vi "Main.vi"() -> ()   [LabVIEW 2020]
doc: "This template is for the Queued Message Handler design pattern.\n\nThe Event Handling Loop generates messages based on user interface actions.\n\nThe Message Handling Loop processes messages generated by the Event Handling Loop, or by other messages. The messages are string values, so new messages can be added easily to the Message Cases case structure in the Message Handling Loop. Each message cluster can also provide an optional value for Message Data, which is a variant that can be converted to whatever message-specific data is required."
uses:
  controls/Parametros.ctl
  controls/UI Data.ctl
  support/Message Queue/Enqueue Message (Single).vi
  <vilib>/Utility/error.llb/Error Cluster From Error Code.vi
  <vilib>/ErrorRing/Error Ring.xnode
  support/Message Queue/Message Queue.lvlib
  support/User Event - Stop/User Event - Stop.lvlib
panel:
  out "Waveform Graph - Dark":dbl[](graph)
  in  "Exit":bool
  in  "Time unit":enum16{"Hours", "Minutes", "Seconds"}(ring)
  in  "Timeout for saving":u32
  in  "Save Switch":bool
  in  "Fecha de inicio":timestamp format="%<%.0X %x>T"
  in  "Graph Button":bool
  in  "Parámetro":T1
  in  "Temperatura carcasa":dbl
  in  "Corriente":dbl
  in  "Voltaje":dbl
  in  "Velocidad del motor":dbl
  in  "Factor de potencia":dbl
  in  "Temperatura balero":dbl
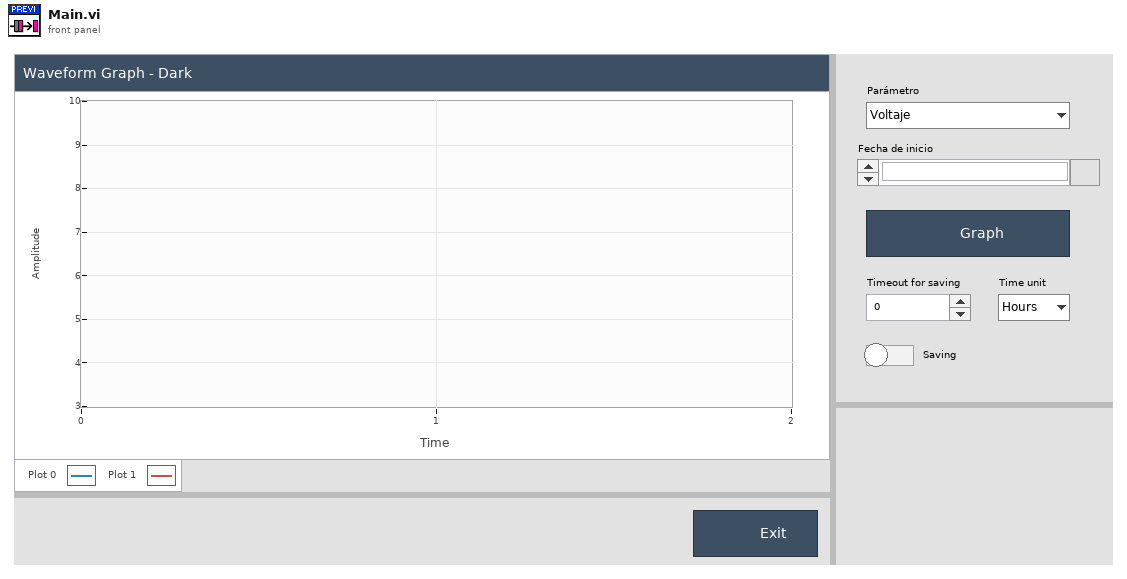
[diagram p1: front panel]
types:
  T1 = typedef "Parametros.ctl" = enum16{"Voltaje", "Corriente", "Temperatura de la carcasa", "Temperatura de balero", "Factor de potencia", "Velocidad de motor"}
  T2 = typedef "UI Data.ctl" = cluster{"Saving":bool, "Exit Button Ref":refnum<vi>, "Time":u32}
  T3 = typedef "Message Queue.lvlib/All Message Queues.ctl" = cluster{"UI":refnum<queue>}
  T4 = cluster{"Timeout for saving":u32, "Time unit":enum16{"Hours", "Minutes", "Seconds"}, "Save Switch":bool}
  T5 = cluster{"Fecha de inicio":timestamp, "Parámetro":T1}
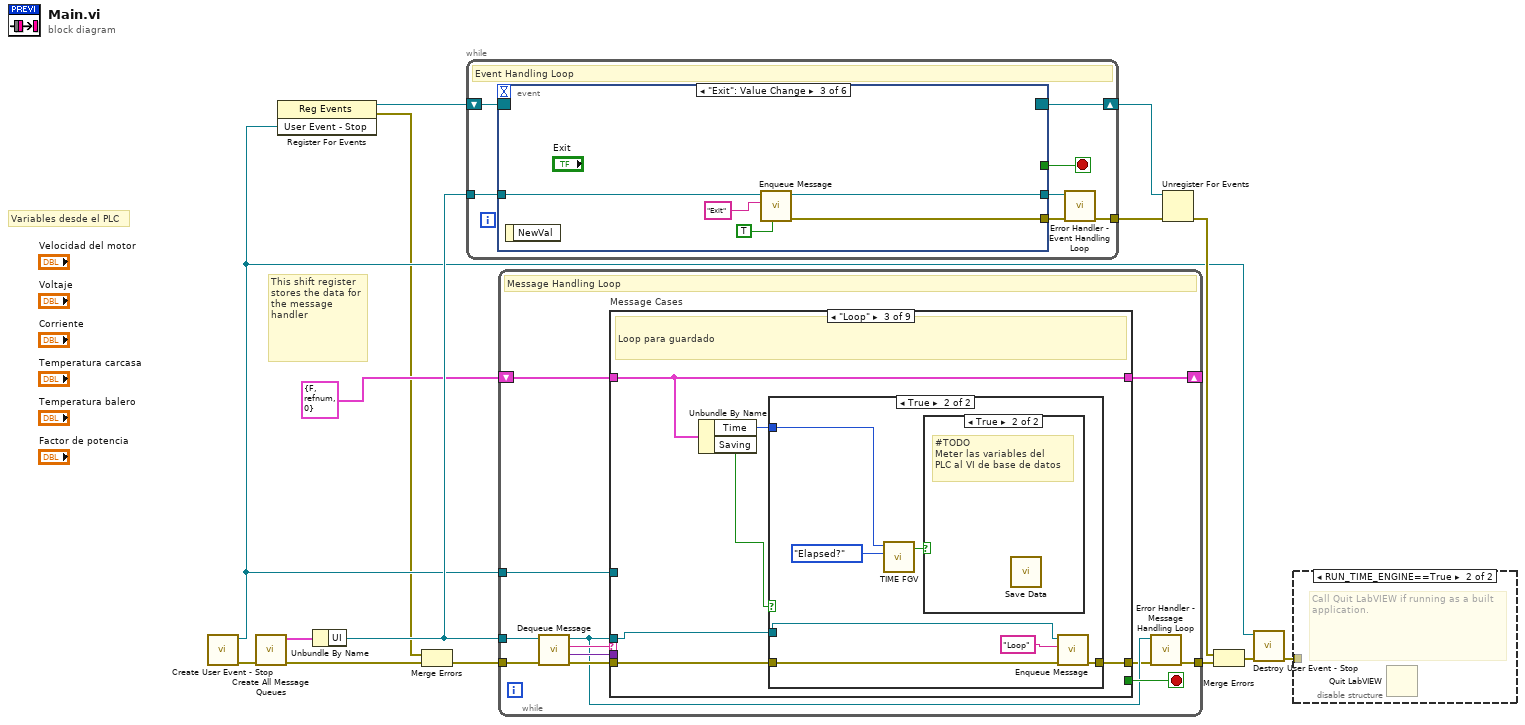
[diagram p0: block diagram]
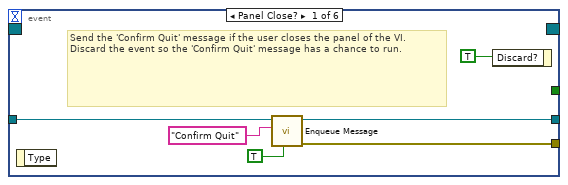
[diagram p3: hidden frame]
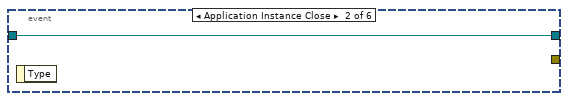
[diagram p4: hidden frame]
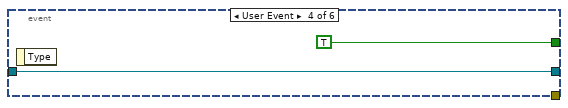
[diagram p5: hidden frame]
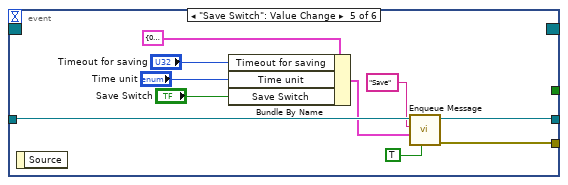
[diagram p6: hidden frame]
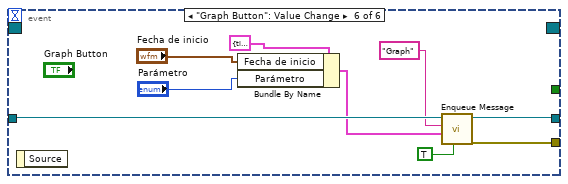
[diagram p7: hidden frame]
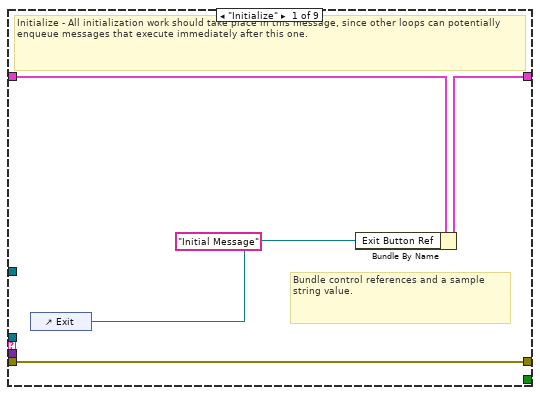
[diagram p8: hidden frame]
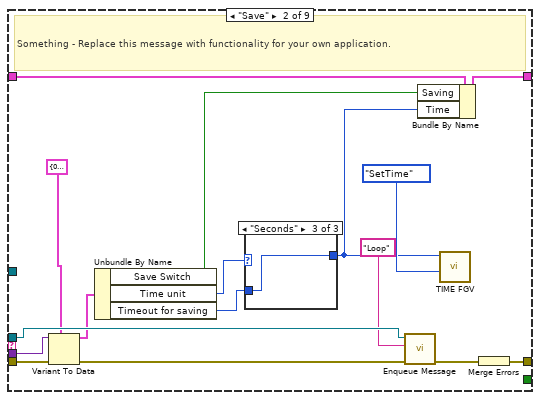
[diagram p9: hidden frame]
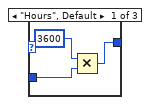
[diagram p10: hidden frame]
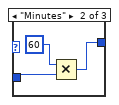
[diagram p11: hidden frame]
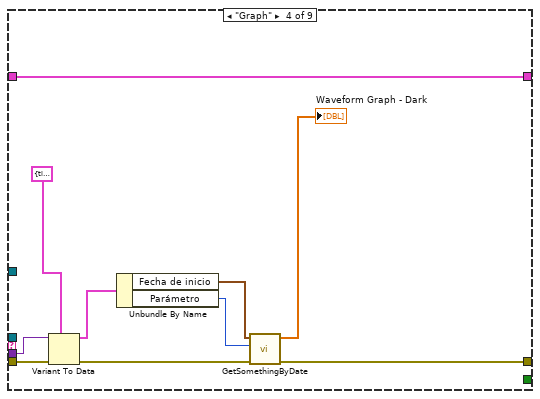
[diagram p14: hidden frame]
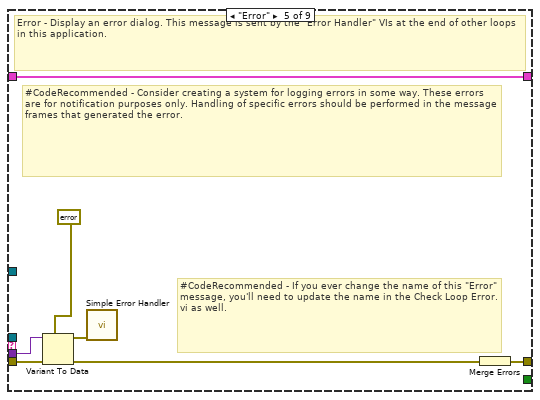
[diagram p15: hidden frame]
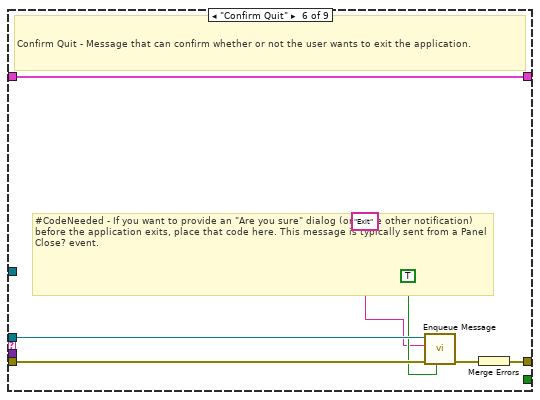
[diagram p16: hidden frame]
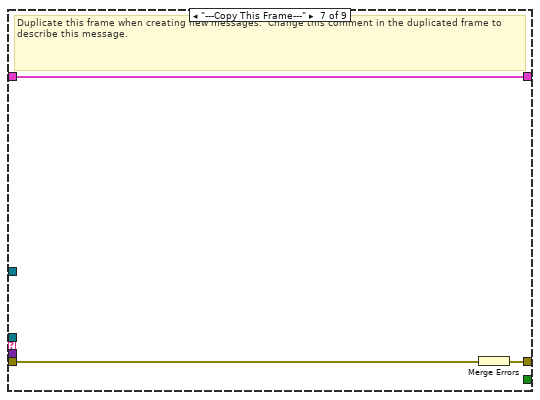
[diagram p17: hidden frame]
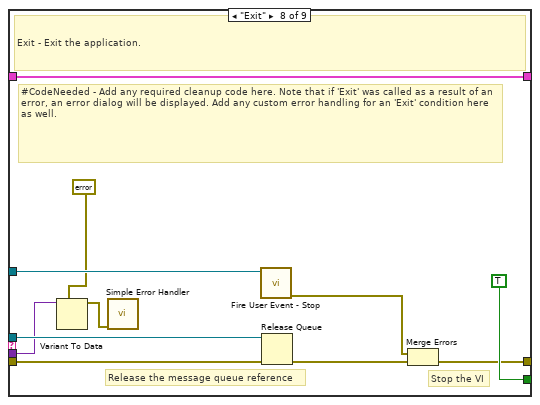
[diagram p18: hidden frame]
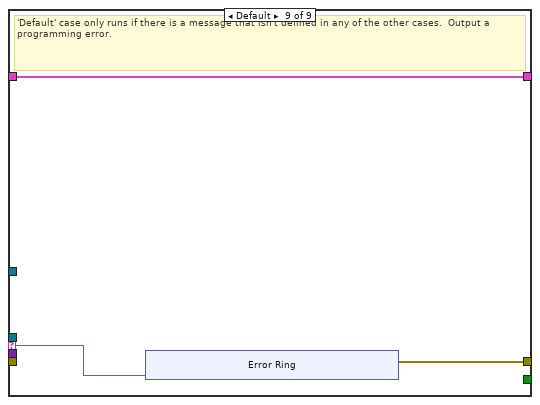
[diagram p19: hidden frame]
diagram:
  # "Variables desde el PLC"
  # "This shift register stores the data for the message handler"
  n1 = call "Create User Event - Stop.vi"() -> ("error out"=w11:errorcluster, "User Event - Stop"=w3:refnum<user-event>)  [unwired: 10 in]
  n2 = call "Create All Message Queues.vi"("error in (no error)"=w11) -> ("error out"=w15:errorcluster, "Message Queues out"=w14:T3)  [unwired: 9 in]
  n3 = register-events(w3) -> (reference out=w4:refnum<event-registration>, error out=w1:errorcluster)  [unwired: 2 in]
  n4 = Unbundle By Name(w14) -> ("UI"=w12:refnum<queue>)
  n5 = Merge Errors(w1, w15) -> (w2:errorcluster)
  n6 = while {
    tunnel: w12 -> [w22]
    shift-right: [w20] -> w8
    shift-left: w4 -> [w21]
    tunnel: [w16] -> w5
    stop <- w18 stop-if-true
    # "Event Handling Loop"
    n7 = event shown="[2] \"Exit\": Value Change" {
      selector: w21 -> [_ _ _ _ _ _]
      dyn-events: [_ _ _ _ _ _] -> w20
      timeout: _ -> [_ _ _ _ _ _]
      tunnel: [_ _ _ TRUE ("Discard?") _ _] -> w18
      tunnel: w22 -> [w27 w29 w34 w36 w46 w53]
      tunnel: [w26 _ w33 _ w44 w54] -> w19
      tunnel: [w25 w29 w32 w36 w45 w55] -> w17
      event Panel Close? {
        # "Send the 'Confirm Quit' message if the user closes the panel of the VI. Discard the event so the 'Confirm Quit' message has a chance to run."
        n8 = event-data() -> ()  [unwired: 1 in, 1 out]
        n9 = call-poly "Enqueue Message.vi"("Priority Message? (F)"=TRUE, "Message"="Confirm Quit", "Message Queue"=w27) -> ("error out"=w26:errorcluster, "dup Message Queue"=w25:refnum<queue>)  [unwired: 7 in]
        n10 = event-data("Discard?"=TRUE) -> ()  [unwired: 1 in, 1 out]
      }
      event Application Instance Close {
        n11 = event-data() -> ()  [unwired: 1 in, 1 out]
      }
      event "Exit": Value Change {
        n12 = event-data() -> ()  [unwired: 1 in, 1 out]
        n13 = call-poly "Enqueue Message.vi"("Priority Message? (F)"=TRUE, "Message"="Exit", "Message Queue"=w34) -> ("error out"=w33:errorcluster, "dup Message Queue"=w32:refnum<queue>)  [unwired: 7 in]
      }
      event User Event {
        n14 = event-data() -> ()  [unwired: 1 in, 1 out]
      }
      event "Save Switch": Value Change {
        n15 = event-data() -> ()  [unwired: 1 in, 1 out]
        n16 = Bundle By Name(cluster=T4 {"Timeout for saving"=0, "Time unit"=enum."Hours", "Save Switch"=FALSE}, "Timeout for saving"="Timeout for saving", "Time unit"="Time unit", "Save Switch"="Save Switch") -> (w38:T4)
        n17 = call-poly "Enqueue Message.vi"("Priority Message? (F)"=TRUE, "Message Data"=w38, "Message"="Save", "Message Queue"=w46) -> ("error out"=w44:errorcluster, "dup Message Queue"=w45:refnum<queue>)  [unwired: 6 in]
      }
      event "Graph Button": Value Change {
        n18 = event-data() -> ()  [unwired: 1 in, 1 out]
        n19 = Bundle By Name(cluster=T5 {"Fecha de inicio"=timestamp(0 s since 1904-01-01), "Parámetro"=enum."Voltaje"}, "Fecha de inicio"="Fecha de inicio", "Parámetro"="Parámetro") -> (w48:T5)
        n20 = call-poly "Enqueue Message.vi"("Priority Message? (F)"=TRUE, "Message Data"=w48, "Message"="Graph", "Message Queue"=w53) -> ("error out"=w54:errorcluster, "dup Message Queue"=w55:refnum<queue>)  [unwired: 6 in]
      }
    }
    n21 = call "Error Handler - Event Handling Loop.vi"("error in (no error)"=w19, "Message Queue"=w17) -> ("dup error in"=w16:errorcluster)  [unwired: 8 in, 1 out]
  }
  n22 = while {
    tunnel: w12 -> [w59]
    shift-right: [w66] -> _
    shift-left: T2 {"Saving"=FALSE, "Exit Button Ref"=refnum, "Time"=0} ("Data Cluster") -> [w67]
    tunnel: w3 -> [w64]
    tunnel: w2 -> [w63]
    tunnel: [w57] -> w13
    stop <- w65 stop-if-true
    # "Message Handling Loop"
    n23 = call "Dequeue Message.vi"("error in (no error)"=w63, "Message Queue"=w59) -> ("error out"=w62:errorcluster, "Message Data"=w60:variant, "Message"=w61:string, "dup Message Queue"=w58:refnum<queue>)  [unwired: 6 in]
    n24 = case "Message Cases" shown="\"Loop\"" w61 {
      selector: w61 -> [_ _ _ _ _ _ _ _ w147]
      tunnel: w58 -> [_ w83 w96 _ _ w128 _ w146 _]
      tunnel: w62 -> [w71 w85 w99 w118 w125 w132 w135 w139 _]
      tunnel: [w71 w86 w100 w109 w119 w130 w133 w142 w148] -> w56
      tunnel: w67 -> [w70 w87 w98 w117 w124 w131 w134 w145 w149]
      tunnel: [w69 w80 w98 w117 w124 w131 w134 w145 w149] -> w66
      tunnel: [_ _ _ _ _ _ _ TRUE _] -> w65
      tunnel: w60 -> [_ w81 _ w116 w123 _ _ w136 _]
      tunnel: w64 -> [_ _ _ _ _ _ _ w141 _]
      frame "Initialize" {
        (unwired) "Initial Message" ("Initial Message")
        # "Bundle control references and a sample string value."
        # "Initialize - All initialization work should take place in this message, since other loops can potentially enqueue messages that execute immediately after this one."
        n25 = control-ref of="Exit"() -> (w68:refnum<vi>)
        n26 = Bundle By Name(cluster=w70, "Exit Button Ref"=w68) -> (w69:T2)
      }
      frame "Save" {
        # "Something - Replace this message with functionality for your own application."
        n27 = Variant To Data(error in=w85, type=T4 {"Timeout for saving"=0, "Time unit"=enum."Hours", "Save Switch"=FALSE}, Variant=w81) -> (data=w77:T4, error out=w82:errorcluster)
        n28 = Unbundle By Name(w77) -> ("Save Switch"=w76:bool, "Time unit"=w75:enum16{"Hours", "Minutes", "Seconds"}, "Timeout for saving"=w74:u32)
        n29 = case shown="\"Seconds\"" w75 {
          tunnel: w74 -> [w89 w93 w94]
          tunnel: [w88 w91 w94] -> w72
          frame "Hours", Default {
            n30 = Multiply(x=u32 3600, y=w89) -> (x*y=w88:u32)
          }
          frame "Minutes" {
            n31 = Multiply(x=u32 60, y=w93) -> (x*y=w91:u32)
          }
          frame "Seconds" {
          }
        }
        n32 = call-poly "Enqueue Message.vi"("error in (no error)"=w82, "Message"="Loop", "Message Queue"=w83) -> ("error out"=w84:errorcluster)  [unwired: 7 in, 1 out]
        n33 = Bundle By Name(cluster=w87, "Saving"=w76, "Time"=w72) -> (w80:T2)
        n34 = call "TIME FGV.vi"("Enum"=enum16{"Elapsed?", "SetTime"}."SetTime", "Time in seconds"=w72) -> ()  [unwired: 9 in, 1 out]
        n35 = Merge Errors(w84) -> (w86:errorcluster)
      }
      frame "Loop" {
        # "Loop para guardado"
        n36 = Unbundle By Name(w98) -> ("Time"=w95:u32, "Saving"=w97:bool)
        n37 = case shown="True" w97 {
          tunnel: [w101 w108] -> w100
          tunnel: w99 -> [w101 w107]
          tunnel: w96 -> [_ w105]
          tunnel: w95 -> [_ w102]
          frame False {
          }
          frame True {
            n38 = call "TIME FGV.vi"("Enum"=enum16{"Elapsed?", "SetTime"}."Elapsed?", "Time in seconds"=w102) -> ("Time Elapsed?"=w103:bool)  [unwired: 9 in]
            n39 = case shown="True" w103 {
              frame False {
              }
              frame True {
                # "#TODO\nMeter las variables del \nPLC al VI de base de datos"
                n40 = call "Save Data.vi"() -> ()  [unwired: 11 in, 1 out]
              }
            }
            n41 = call-poly "Enqueue Message.vi"("error in (no error)"=w107, "Message"="Loop", "Message Queue"=w105) -> ("error out"=w108:errorcluster)  [unwired: 7 in, 1 out]
          }
        }
      }
      frame "Graph" {
        n42 = Variant To Data(error in=w118, type=T5 {"Fecha de inicio"=timestamp(0 s since 1904-01-01), "Parámetro"=enum."Voltaje"}, Variant=w116) -> (data=w114:T5, error out=w110:errorcluster)
        n43 = Unbundle By Name(w114) -> ("Fecha de inicio"=w113:timestamp, "Parámetro"=w112:T1)
        n44 = call "GetSomethingByDate.vi"("error in (no error)"=w110, "Parámetro"=w112, "Time Stamp"=w113) -> ("error out"=w109:errorcluster, "Result Set"=→"Waveform Graph - Dark":dbl[])  [unwired: 7 in]
      }
      frame "Error" {
        # "#CodeRecommended - If you ever change the name of this \"Error\" message, you'll need to update the name in the Check Loop Error.vi as well."
        # "#CodeRecommended - Consider creating a system for logging errors in some way. These errors are for notification purposes only. Handling of specific errors should be performed in the message frames that generated the error."
        # "Error - Display an error dialog. This message is sent by the \"Error Handler\" VIs at the end of other loops in this application."
        n45 = Variant To Data(error in=w125, type=errorcluster {"status"=FALSE, "code"=0, "source"=""} ("error constant"), Variant=w123) -> (data=w121:errorcluster, error out=w120:errorcluster)
        n46 = call <vilib>:"Simple Error Handler.vi"("error in (no error)"=w121) -> ()  [unwired: 4 in, 5 out]
        n47 = Merge Errors(w120) -> (w119:errorcluster)
      }
      frame "Confirm Quit" {
        # "#CodeNeeded - If you want to provide an \"Are you sure\" dialog (or some other notification) before the application exits, place that code here. This message is typically sent from a Panel Close? event."
        # "Confirm Quit - Message that can confirm whether or not the user wants to exit the application."
        n48 = call-poly "Enqueue Message.vi"("Priority Message? (F)"=TRUE, "error in (no error)"=w132, "Message"="Exit", "Message Queue"=w128) -> ("error out"=w129:errorcluster)  [unwired: 6 in, 1 out]
        n49 = Merge Errors(w129) -> (w130:errorcluster)
      }
      frame "---Copy This Frame---" {
        # "Duplicate this frame when creating new messages.  Change this comment in the duplicated frame to describe this message."
        n50 = Merge Errors(w135) -> (w133:errorcluster)
      }
      frame "Exit" {
        # "Stop the VI"
        # "Release the message queue reference"
        # "#CodeNeeded - Add any required cleanup code here. Note that if 'Exit' was called as a result of an error, an error dialog will be displayed. Add any custom error handling for an 'Exit' condition here as well."
        # "Exit - Exit the application."
        n51 = Variant To Data(type=errorcluster {"status"=FALSE, "code"=0, "source"=""} ("error constant"), Variant=w136) -> (data=w137:errorcluster)  [unwired: 1 in, 1 out]
        n52 = call <vilib>:"Simple Error Handler.vi"("error in (no error)"=w137) -> ()  [unwired: 4 in, 5 out]
        n53 = call "Fire User Event - Stop.vi"("User Event - Stop"=w141) -> ("error out"=w140:errorcluster)  [unwired: 10 in]
        n54 = Release Queue(queue=w146, error in (no error)=w139) -> (error out=w143:errorcluster)  [unwired: 1 in, 2 out]
        n55 = Merge Errors(w140, w143) -> (w142:errorcluster)
      }
      frame Default {
        # "'Default' case only runs if there is a message that isn't defined in any of the other cases.  Output a programming error."
        n56 = xnode "Error Ring"("parameter 0"=w147) -> ("error out"=w148:errorcluster)
      }
    }
    n57 = call "Error Handler - Message Handling Loop.vi"("error in (no error)"=w56, "Message Queue"=w58) -> ("dup error in"=w57:errorcluster)  [unwired: 8 in, 1 out]
  }
  n58 = Unregister For Events(event registration refnum=w8, error in=w5) -> (error out=w9:errorcluster)
  n59 = Merge Errors(w9, w13) -> (w10:errorcluster)
  n60 = call "Destroy User Event - Stop.vi"("error in (no error)"=w10, "User Event - Stop"=w3) -> ("error out"=w6:errorcluster)  [unwired: 9 in]
  n61 = disable-structure shown="RUN_TIME_ENGINE==True" {
    disable-tunnel: w6 -> [_ _]
    frame condition #0 (active) {
    }
    frame condition #1 {
      # "Call Quit LabVIEW if running as a built application."
      n62 = Quit LabVIEW() -> ()  [unwired: 1 in]
    }
  }
